vi "Vol-Determine data type and ROI ID.vi"() -> (0 "ROI ID Enum":T1, 1 "Valid path":bool, 2 "Functional data type":T2, 3 "Valid data type":bool)   [LabVIEW 2020]
uses:
  Typedefs/Functional data family.ctl
  Typedefs/ROI ID Enum.ctl
  Timelapse Viewer/Globals/gl_Time series viewer globals.vi
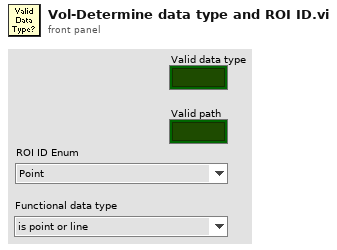
[diagram p1: front panel]
types:
  T1 = typedef "ROI ID Enum.ctl" = enum16{"Point", "MiniScan", "Comp. MiniScan", "Rectangle", "Comp. volume", "Arb. plane point", "None"}
  T2 = typedef "Functional data family.ctl" = enum16{"is point or line", "is surface or volume"}
  T3 = typedef "Time series viewer refs.ctl" = cluster{"This VI":refnum<vi>, "Image control":refnum<vi>, "AVI Mode ind":refnum<vi>, "Play":refnum<vi>, "Stop":refnum<vi>, "Back":refnum<vi>, "Scrollbar":refnum<vi>, "Video length info":refnum<vi>, "Expected speed values":refnum<vi>, "Intensity":refnum<vi>, "Path":refnum<vi>, "Selection sliders":refnum<vi>, "Speed Graph ref":refnum<vi>, "Frame rate set (fps)":refnum<vi>, "Number of rows to generate":refnum<vi>, "VL Image Array":refnum<vi>, "Image Scrollbar":refnum<vi>, "Channel to load":refnum<vi>, "Colour":refnum<vi>}
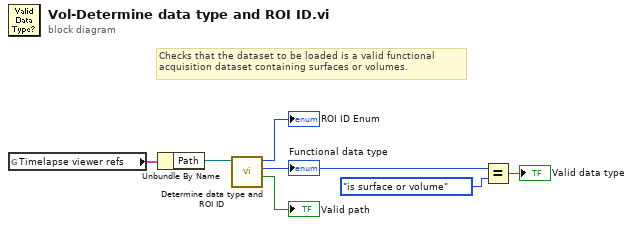
[diagram p0: block diagram]
diagram:
  # "Checks that the dataset to be loaded is a valid functional acquisition dataset containing surfaces or volumes."
  n1 = global read "gl_Time series viewer globals.vi" "Timelapse viewer refs"() -> (w7:T3)
  n2 = Unbundle By Name(w7) -> ("Path"=w6:refnum<vi>)
  n3 = call "Determine data type and ROI ID.vi"("Dataset path"=w6) -> ("Valid path"=→"Valid path":bool, "Functional data type"=w4:T2, "ROI ID Enum"=→"ROI ID Enum":T1)  [unwired: 8 in]
  "Functional data type" <- w4
  n4 = Equal?(x=w4, y=Functional_data_family."is surface or volume") -> (x = y?=→"Valid data type":bool)
